vi "Wheelspeed.vi"(1 "Max Speed":dbl, 2 "Yi(t)":dbl, 3 "H":dbl, 4 "V":dbl, 5 "U":dbl) -> (0 "Wheelspeed":dbl)   [LabVIEW 2012]
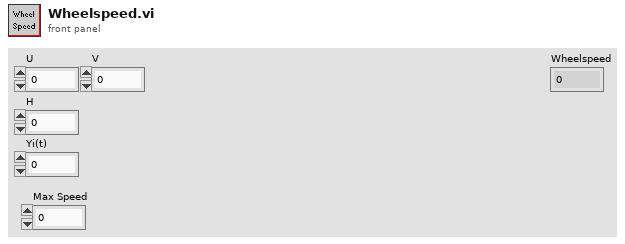
[diagram p1: front panel]
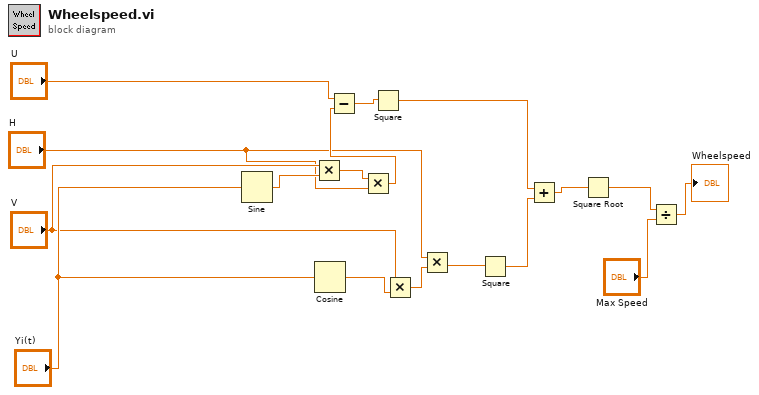
[diagram p0: block diagram]
diagram:
  n1 = Sine(x="Yi(t)") -> (sin(x)=w17:dbl)
  n2 = Multiply(x="V", y=w17) -> (x*y=w16:dbl)
  n3 = Cosine(x="Yi(t)") -> (cos(x)=w11:dbl)
  n4 = Multiply(x=w16, y="H") -> (x*y=w15:dbl)
  n5 = Subtract(x="U", y=w15) -> (x-y=w13:dbl)
  n6 = Square(x=w13) -> (x^2=w5:dbl)
  n7 = Multiply(x="V", y=w11) -> (x*y=w9:dbl)
  n8 = Multiply(x="H", y=w9) -> (x*y=w7:dbl)
  n9 = Square(x=w7) -> (x^2=w6:dbl)
  n10 = Add(x=w5, y=w6) -> (x+y=w4:dbl)
  n11 = Square Root(x=w4) -> (sqrt(x)=w3:dbl)
  n12 = Divide(x=w3, y="Max Speed") -> (x/y=→"Wheelspeed":dbl)
